vi "LoadNewGraph_LS1.vi"(5 "MainGraphQ":refnum<queue>, 7 "GraphEvent":refnum<user-event>, 8 "ErrIn(No Err)":errorcluster caption="entrée d'erreur (pas d'erreur)", 9 "GraphNumber":i32, 10 "FAIndex":i32, 11 "Graph_FA":refnum<vi>[](array[refnum])) -> (0 "ErrOut":errorcluster caption="sortie d'erreur", 1 "Graph":refnum<vi>, 2 "GraphQRef":refnum<queue>, 3 "Graph_FA Out":refnum<vi>[](array[refnum]))   [LabVIEW 2019]
uses:
  GraphQData.ctl
  Interface Class/Interface.lvclass
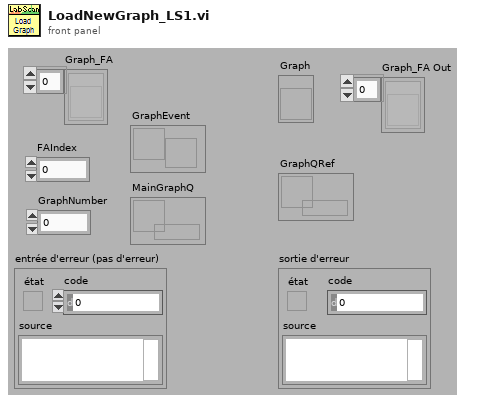
[diagram p1: front panel]
types:
  T1 = enum16{"Répertoire du VI actuel", "Répertoire du parent 1", "Répertoire du parent 2", "Répertoire du parent 3"}
  T2 = enum32{"Invalid", "Standard", "Closed", "Hidden", "Minimized", "Maximized"}
  T3 = typedef "Interface.lvclass/GraphQData.ctl" = cluster{"Message":string, "Data":variant, "Time":i32, "GraphData":cluster{dbl[], dbl[]}[]}
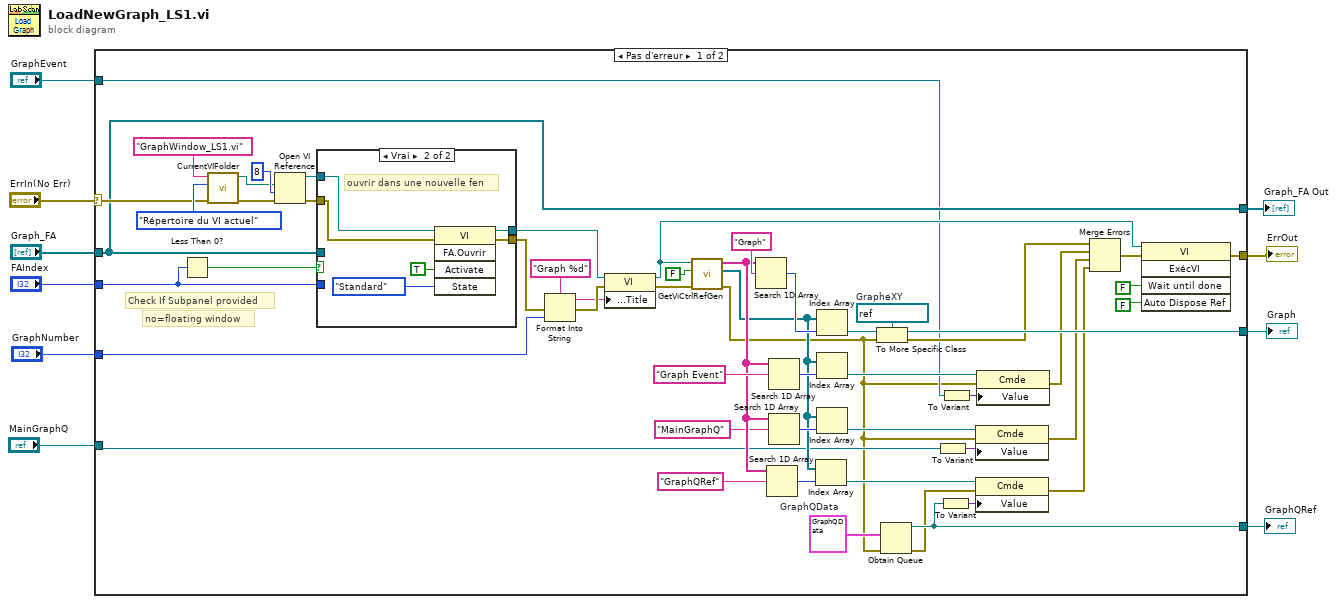
[diagram p0: block diagram]
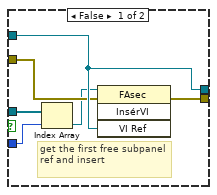
[diagram p2: hidden frame]
diagram:
  n1 = case shown="Pas d'erreur" "ErrIn(No Err)" {
    selector: "ErrIn(No Err)" -> [w61 w77]
    tunnel: [w28 w77] -> w9
    tunnel: "Graph_FA" -> [w42 w76]
    tunnel: [w42 w76] -> w7
    tunnel: [w54 _] -> w6
    tunnel: "FAIndex" -> [w49 _]
    tunnel: "GraphNumber" -> [w46 _]
    tunnel: [w33 _] -> w3
    tunnel: "GraphEvent" -> [w24 _]
    tunnel: "MainGraphQ" -> [w17 _]
    frame No Error {
      w13 = T3 {"Message"="", "Data"=variant, "Time"=0, "GraphData"=[]}  # GraphQData
      w53 = refnum<vi> refnum  # GrapheXY
      # "no=floating window"
      # "Check If Subpanel provided"
      n2 = Less Than 0?(x=w49) -> (x < 0?=w48:bool)
      n3 = call <userlib>:"CurrentVIFolder.vi"("error in (no error)"=w61, "Source"=T1."Répertoire du VI actuel", "NomFichier"="GraphWindow_LS1.vi") -> ("error out"=w63:errorcluster, "Chemin"=w31:path)  [unwired: 6 in, 1 out]
      n4 = Open VI Reference(vi path=w31, options=8, error in (no error)=w63) -> (vi reference=w52:refnum<vi>, error out=w59:errorcluster)  [unwired: 3 in]
      n5 = case shown="Vrai" w48 {
        tunnel: w59 -> [w65 w70]
        tunnel: w52 -> [w66 w71]
        tunnel: [w69 w75] -> w25
        tunnel: w42 -> [w68 _]
        tunnel: [w66 w74] -> w30
        tunnel: w49 -> [w67 _]
        frame False {
          # "get the first free subpanel ref and insert"
          n6 = Index Array(array=w68, index=w67) -> (element=w64:refnum<vi>)
          n7 = invoke class="FAsec" method="InsérVI"(reference=w64, error in=w65, "VI Ref"=w66) -> (error out=w69:errorcluster)  [unwired: 1 in, 3 out]
        }
        frame True {
          # "ouvrir dans une nouvelle fen"
          n8 = invoke class="VI" method="FA.Ouvrir"(reference=w71, error in=w70, "Activate"=TRUE ("Activer ?"), "State"=T2."Standard" ("État")) -> (reference out=w74:refnum<vi>, error out=w75:errorcluster)  [unwired: 1 in, 3 out]
        }
      }
      n9 = Format Into String(format string="Graph %d" ("chaîne de format"), error in=w25, w46) -> (resulting string=w26:string, error out=w44:errorcluster)  [unwired: 1 in]
      n10 = property class="VI"(reference=w30, error in=w44, "Front Panel.Title"=w26) -> (reference out=w27:refnum<vi>, error out=w47:errorcluster)
      n11 = call <userlib>:"GetViCtrlRefGen.vi"("ErrorIn(No Error)"=w47, "InclTabCTrl"=FALSE, "VIRef"=w27) -> ("sortie d'erreur"=w11:errorcluster, "ControlsRefs"=w21:refnum<vi>[], "ControlsNames"=w22:string[])  [unwired: 6 in]
      n12 = Search 1D Array(1D array=w22, element="Graph" ("élément")) -> (index of element=w56:i32)  [unwired: 1 in]
      n13 = Search 1D Array(1D array=w22, element="GraphQRef" ("élément")) -> (index of element=w36:i32)  [unwired: 1 in]
      n14 = Search 1D Array(1D array=w22, element="Graph Event" ("élément")) -> (index of element=w40:i32)  [unwired: 1 in]
      n15 = Search 1D Array(1D array=w22, element="MainGraphQ" ("élément")) -> (index of element=w23:i32)  [unwired: 1 in]
      n16 = Index Array(array=w21, index=w36) -> (element=w34:refnum<vi>)
      n17 = Index Array(array=w21, index=w56) -> (element=w55:refnum<vi>)
      n18 = Index Array(array=w21, index=w40) -> (element=w39:refnum<vi>)
      n19 = Index Array(array=w21, index=w23) -> (element=w19:refnum<vi>)
      n20 = To More Specific Class(target class=w53, reference=w55, error in=w11) -> (specific class reference=w54:refnum<vi>, error out=w43:errorcluster)
      n21 = Obtain Queue(element data type=w13, error in (no error)=w11) -> (queue out=w33:refnum<queue>, error out=w32:errorcluster)  [unwired: 3 in, 1 out]
      n22 = To Variant(anything=w17) -> (Variant=w20:variant)
      n23 = To Variant(anything=w33) -> (Variant=w14:variant)
      n24 = To Variant(anything=w24) -> (Variant=w38:variant)
      n25 = property class="Cmde"(reference=w19, error in=w11, "Value"=w20) -> (error out=w16:errorcluster)  [unwired: 1 out]
      n26 = property class="Cmde"(reference=w34, error in=w32, "Value"=w14) -> (error out=w15:errorcluster)  [unwired: 1 out]
      n27 = property class="Cmde"(reference=w39, error in=w11, "Value"=w38) -> (error out=w37:errorcluster)  [unwired: 1 out]
      n28 = Merge Errors(w43, w37, w16, w15) -> (w29:errorcluster)
      n29 = invoke class="VI" method="ExécVI"(reference=w27, error in=w29, "Wait until done"=FALSE ("Attendre la fin"), "Auto Dispose Ref"=FALSE ("Supprimer la référence automatiquement")) -> (error out=w28:errorcluster)  [unwired: 1 in, 4 out]
    }
    frame Error {
    }
  }
  "ErrOut" <- w9
  "Graph_FA Out" <- w7
  "Graph" <- w6
  "GraphQRef" <- w3
